vi "RT_stagectrl_readIFO_3levelramp_Nov4.vi"() -> ()   [LabVIEW 2019]
uses:
  <vilib>/Platform/TimedLoop/XDataNode/timing_clust.ctl
  <vilib>/Platform/TimedLoop/XDataNode/nitl_modes.ctl
  <vilib>/Platform/TimedLoop/XDataNode/wakeup.ctl
  <vilib>/FPGAPlugInAG/myRIO-1900/niLvFpga_Open_myRIO-1900.vi
  <vilib>/rvi/interface/common/dynamic/niFpgaDynamicAddResources.vi
  <vilib>/Utility/error.llb/Error Cluster From Error Code.vi
  <vilib>/rvi/errors/niLvFpgaAdjustHostInterfaceError.vi
  <vilib>/rvi/interface/nirviOpenFPGA/nirviOpenFPGA.xnode
  FPGA Bitfiles/studentchallenge_FPGATarget_FPGA1RADC1WDAC2A_R8uuw9uWLNg.lvbitx
  <vilib>/platform/TimedLoop/XDataNode/XDataNode.xnode
  <vilib>/rvi/interface/nirviReadWriteControl/nirviReadWriteControl.xnode
  NiFpgaLv.dll
  <vilib>/rvi/interface/Simulation/niFpgaSimulationCallBeginRW.vi
  <vilib>/Platform/TimedLoop/XDataNode/XDNodeRunTimeDep.lvlib
panel:
  in  "Stop":bool
  in  "P":dbl=2.0
  in  "I":dbl=0.005
  in  "D":dbl
  out "Control voltage":dbl=-0.4460961993175754 format="%#_3f"
  out "late?":bool
  out "?":cluster{"profile des(mm)":dbl, dbl, dbl}(graph)
  in  "Stage loop time (us)":i64=700
  out "Vp":dbl=-0.052695520808333285 format="%#_3g"
  out "Vi":dbl=0.4987253915842921 format="%#_3g"
  out "Vd":dbl format="%#_3g"
  out "profile des(mm)":dbl=1.6059943214036447
  in  "Profile track":bool
  in  "dt":i64=100
  in  "IFO loop time (us)":i64=70
  out "late? 2":bool
  out "IFO (um)":dbl
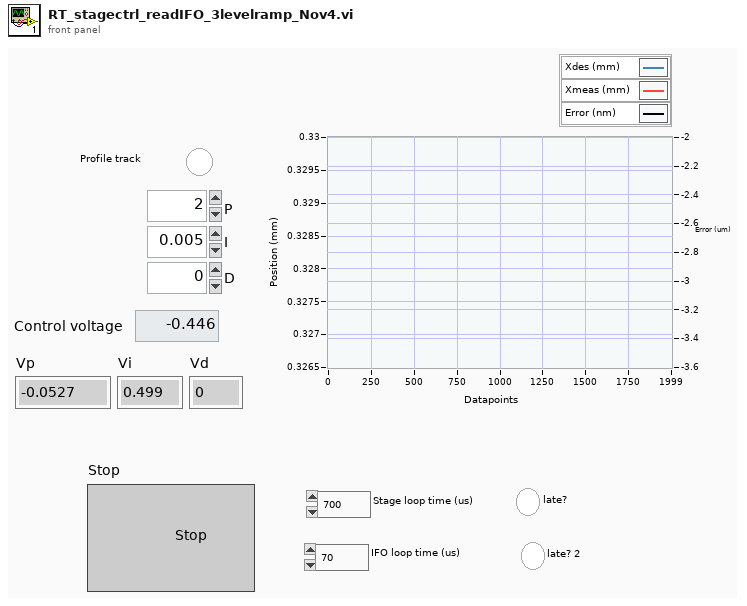
[diagram p1: front panel]
types:
  T1 = typedef "XDNodeRunTimeDep.lvlib/timing_clust.ctl" = cluster{"Expected End [f-1]":u64, "Actual End [f-1]":u64, "Finished Late? [f-1]":bool, "Expected End [i-1]":u64, "Actual End [i-1]":u64, "Finished Late? [i-1]":bool, "Expected Start [i]":u64, "Actual Start [i]":u64, "Expected Start [f]":u64, "Actual Start [f]":u64, "Source Name":string, "Structure Name":string, "Period":i64, "Deadline":i64, "Offset":i64, "Start":i64, "Priority":i32, "Timeout":i32, "Mode":T2, "Wakeup Reason":T3, "Error":errorcluster, "Source Type":string, "Secondary Source Type":string, "Global End Time":u64, "Global Start Time":u64, "Frame Duration":u64, "Iteration Duration":u64, "Assigned CPU":i32, "I/O Scan Engine Mode":u32}
  T2 = typedef "XDNodeRunTimeDep.lvlib/nitl_modes.ctl" = enum32{"No Change", "Process missed periods, maintain original phase", "Discard missed periods, maintain original phase", "Process missed periods, ignore original phase", "Discard missed periods, ignore original phase"}
  T3 = typedef "XDNodeRunTimeDep.lvlib/wakeup.ctl" = enum32{"Normal", "Aborted", "Asynchronous wakeup", "Timing source error", "Timed loop error", "Timeout"}
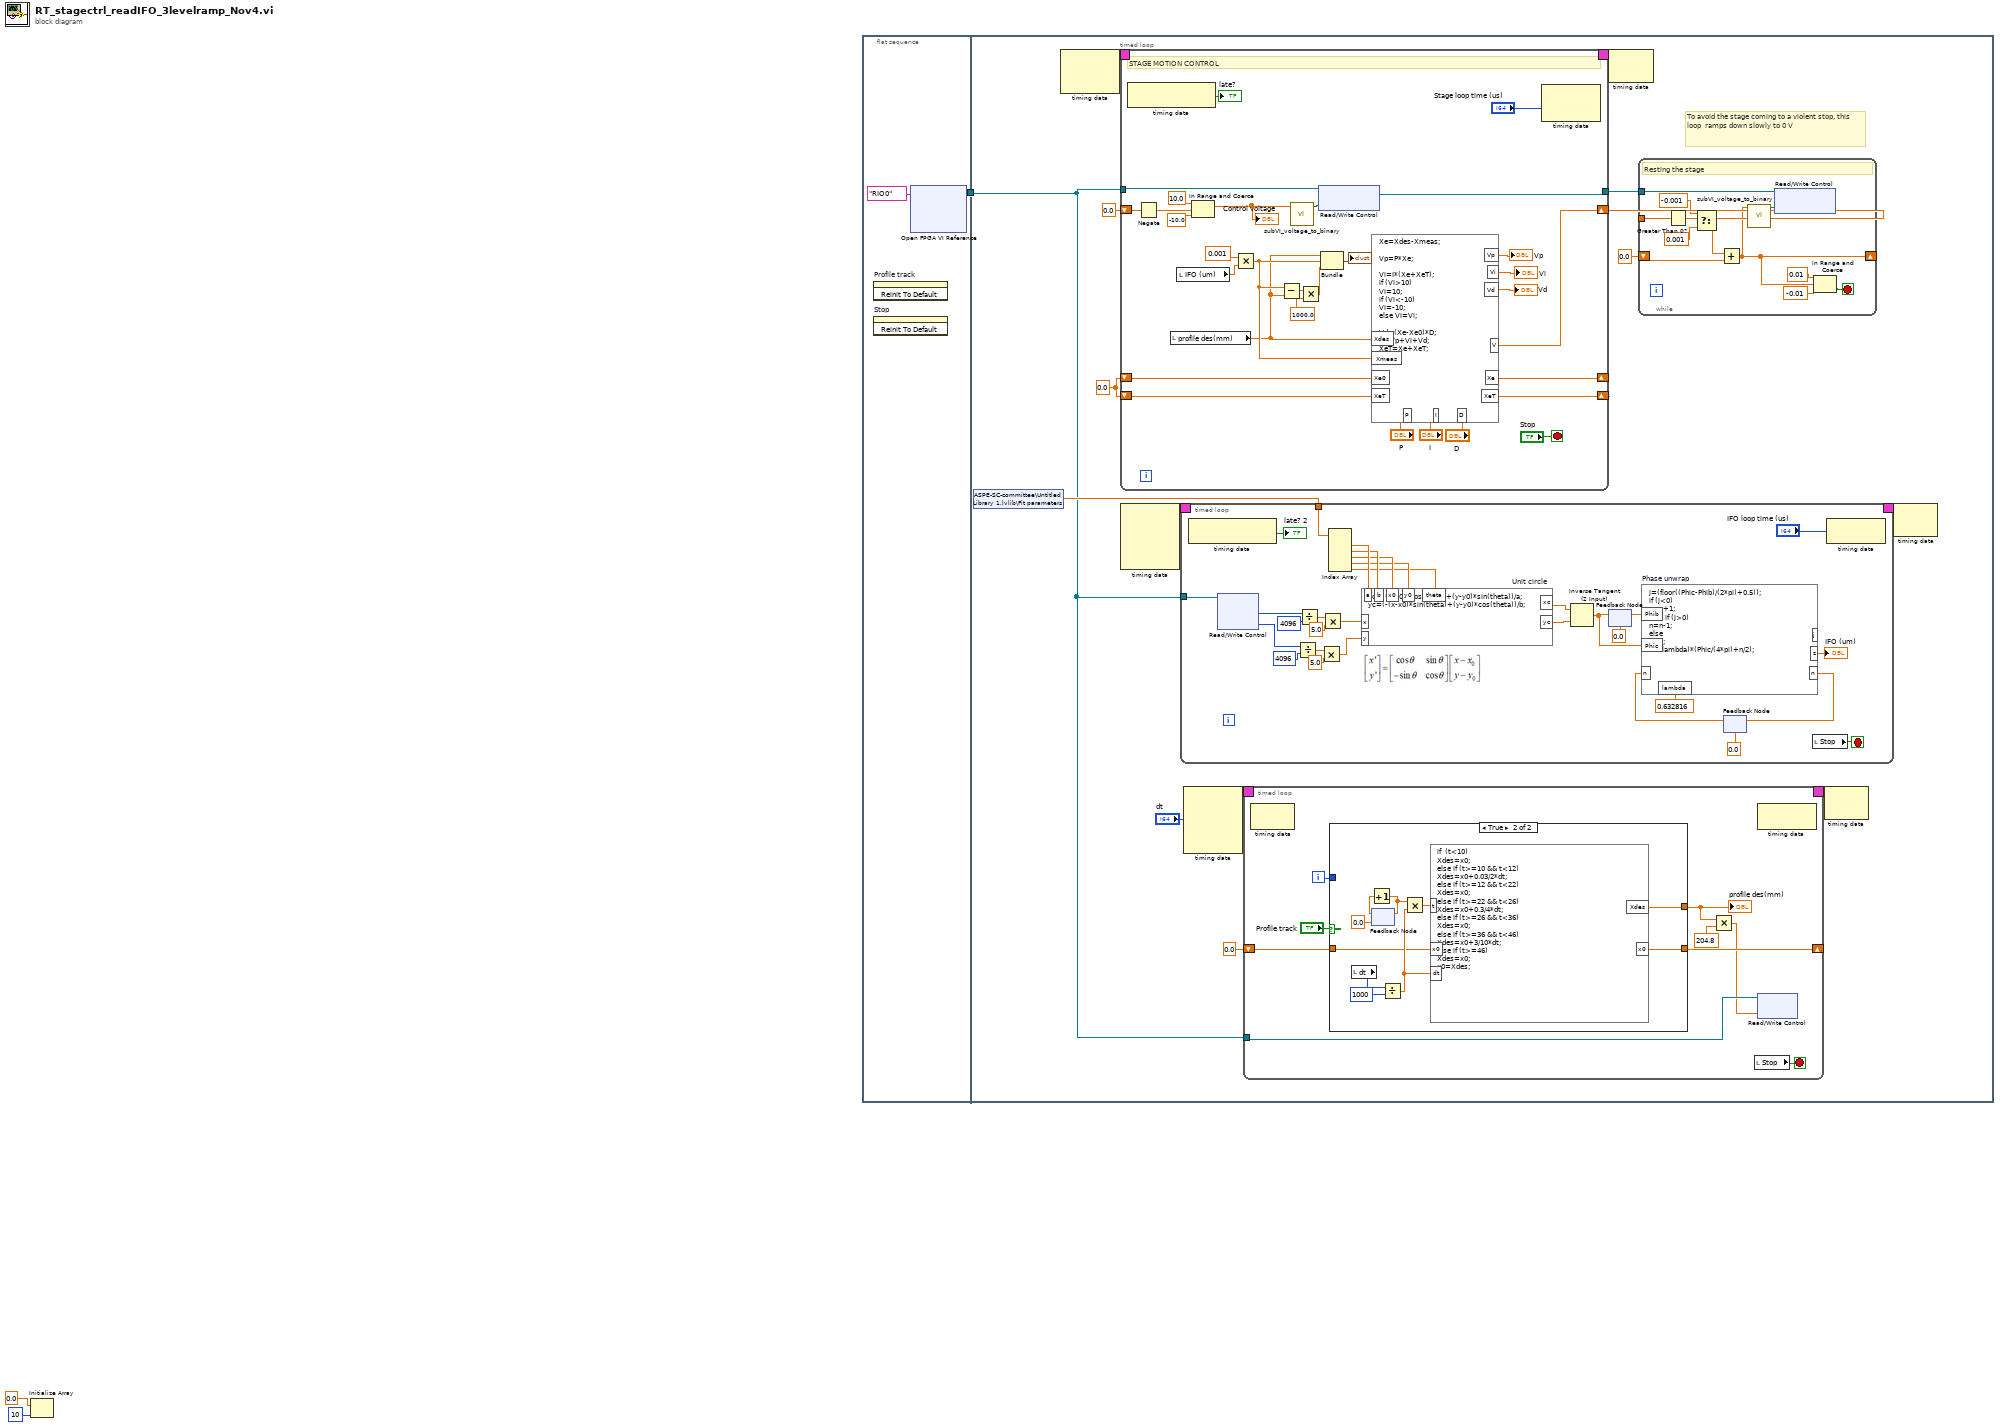
[diagram p0: block diagram]
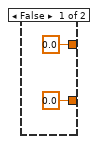
[diagram p2: hidden frame]
diagram:
  n1 = Initialize Array(0.0 ("element"), 10 ("dimension size")) -> ()  [unwired: 1 out]
  n2 = flat-sequence {
    tunnel: [w4] -> w1
    tunnel: w1 -> [w6]
    frame #0 {
      n3 = invoke on="Profile track" class="Bool (strict)" method="Reinit To Default"() -> ()  [unwired: 3 in, 3 out]
      n4 = invoke on="Stop" class="Bool (strict)" method="Reinit To Default"() -> ()  [unwired: 3 in, 3 out]
      n5 = xnode "Open FPGA VI Reference"("resource name"=tag "RIO0") -> ("FPGA VI Reference Out"=w4:refnum<k20>)  [unwired: 1 in, 1 out]
    }
    frame #1 {
      w13 = 0.0 ("Xe")
      # "To avoid the stage coming to a violent stop, this loop  ramps down slowly to 0 V"
      n6 = shared-variable "ASPE-SC-committee\\Untitled Library 1.lvlib\\Fit parameters"() -> (w10:dbl[])  [unwired: 1 in, 1 out]
      n7 = node-c288() -> (w20:T1)  [unwired: 2 in]
      n8 = timed-loop {
        timing: w20 -> [_]
        timing-out: [_] -> w19
        tunnel: [w114] -> w14
        tunnel: w6 -> [w101]
        shift-right: [w112] -> _
        shift-left: w13 -> [w111]
        shift-right: [w110] -> _
        shift-left: w13 -> [w109]
        shift-right: [w88] -> w9
        shift-left: 0.0 ("V") -> [w85]
        stop <- "Stop" stop-if-true
        # "STAGE MOTION CONTROL"
        n9 = node-c288() -> (→"late?":bool)  [unwired: 1 in]
        n10 = Negate(x=w85) -> (-x=w102:dbl)
        n11 = local read "profile des(mm)"() -> (w95:dbl)
        n12 = local read "IFO (um)"() -> (w99:dbl)
        n13 = In Range and Coerce(upper limit=10.0, x=w102, lower limit=-10.0) -> (coerced(x)=w86:dbl)  [unwired: 1 out]
        "Control voltage" <- w86
        n14 = Multiply(x=0.001, y=w99) -> (x*y=w96:dbl)
        n15 = Subtract(x=w96, y=w95) -> (x-y=w94:dbl)
        n16 = call "subVI_voltage_to_binary.vi"("voltage"=w86) -> ("binary"=w100:bool[])  [unwired: 10 in]
        n17 = Multiply(x=w94, y=1000.0) -> (x*y=w87:dbl)
        n18 = xnode "Read/Write Control"("FPGA VI Reference In"=w101, "DAC 1 write"=w100) -> ("FPGA VI Reference Out"=w114:refnum<k20>)  [unwired: 1 in, 1 out]
        n19 = Bundle("profile des(mm)"=w95, w96, w87) -> (→"?":cluster{"profile des(mm)":dbl, dbl, dbl})  [unwired: 1 in]
        n20 = formula code="Xe=Xdes-Xmeas;\n\nVp=P*Xe;\n\nVi=I*(Xe+XeT);\nif (Vi>10)\nVi=10;\nif (Vi<-10)\nVi=-10;\nelse Vi=Vi;\n\nVd=(Xe-Xe0)*D;\nV=Vp+Vi+Vd;\nXeT=Xe+XeT;"("Xdes"=w95, "Xmeas"=w96, "Xe0"=w111, "XeT"=w109, "P"="P", "I"="I", "D"="D") -> ("Xe"=w112:dbl, "V"=w88:dbl, "XeT"=w110:dbl, "Vp"=→"Vp":dbl, "Vi"=→"Vi":dbl, "Vd"=→"Vd":dbl)
        n21 = node-c288("Stage loop time (us)") -> ()  [unwired: 1 in, 1 out]
      }
      n22 = node-c288() -> (w16:T1)  [unwired: 4 in]
      n23 = timed-loop {
        timing: w16 -> [_]
        timing-out: [_] -> w15
        tunnel: w10 -> [w25]
        tunnel: w6 -> [w22]
        stop <- w23 stop-if-true
        n24 = node-c288() -> (→"late? 2":bool)  [unwired: 1 in]
        n25 = xnode "Read/Write Control"("FPGA VI Reference In"=w22) -> ("PD1"=w46:u16, "PD2"=w39:u16)  [unwired: 1 in, 2 out]
        n26 = Divide(x=w39, y=u16 4096) -> (x/y=w41:dbl)
        n27 = Divide(x=w46, y=u16 4096) -> (x/y=w44:dbl)
        n28 = Multiply(x=w41, y=5.0) -> (x*y=w37:dbl)
        n29 = Multiply(x=w44, y=5.0) -> (x*y=w42:dbl)
        n30 = Index Array(array=w25) -> (element #1=w36:dbl, element #2=w35:dbl, element #3=w34:dbl, element #4=w33:dbl, element #5=w32:dbl)  [unwired: 5 in]
        n31 = formula code="xc=((x-x0)*cos(theta)+(y-y0)*sin(theta))/a;\nyc=(-(x-x0)*sin(theta)+(y-y0)*cos(theta))/b;" "Unit circle"("a"=w36, "b"=w35, "x0"=w34, "y0"=w33, "theta"=w32, "x"=w42, "y"=w37) -> ("yc"=w49:dbl, "xc"=w50:dbl)
        n32 = Inverse Tangent (2 Input)(1:w49, 2:w50) -> (0:w28:dbl)
        n33 = feedback #1(0.0) -> (w29:dbl)
        n34 = feedback-in #1(w28) -> ()
        n35 = feedback #2(0.0 ("j")) -> (w30:dbl)
        n36 = formula code="j=(floor((Phic-Phib)/(2*pi)+0.5));\nif (j<0)\nn=n+1;\nelse if (j>0)\nn=n-1;\nelse\nn=n;\nz=(lambda)*(Phic/(4*pi)+n/2);" "Phase unwrap"("Phic"=w28, "Phib"=w29, "n"=w30, "lambda"=0.632816 ("input variable")) -> ("n"=w27:dbl, "z"=→"IFO (um)":dbl)  [unwired: 1 out]
        n37 = feedback-in #2(w27) -> ()
        n38 = local read "Stop"() -> (w23:bool)
        n39 = node-c288("IFO loop time (us)") -> ()  [unwired: 1 out]
      }
      n40 = node-c288("dt") -> (w18:T1)  [unwired: 3 in]
      n41 = timed-loop {
        timing: w18 -> [_]
        timing-out: [_] -> w17
        shift-right: [w66] -> _
        shift-left: 0.0 ("x0") -> [w65]
        tunnel: w6 -> [w61]
        i -> [w63]
        stop <- w62 stop-if-true
        n42 = node-c288() -> ()  [unwired: 1 in, 1 out]
        n43 = case shown="True" "Profile track" {
          tunnel: [0.0 ("x0") w75] -> w66
          tunnel: w65 -> [_ w74]
          tunnel: [0.0 ("Xdes") w69] -> w58
          tunnel: w63 -> [_ _]
          frame False {
          }
          frame True {
            n44 = local read "dt"() -> (w78:i64)
            n45 = feedback #3(0.0) -> (w71:dbl)
            n46 = Increment(x=w71) -> (x+1=w72:dbl)
            n47 = feedback-in #3(w72) -> ()
            n48 = Divide(x=w78, y=i64 1000) -> (x/y=w76:dbl)
            n49 = Multiply(x=w72, y=w76) -> (x*y=w73:dbl)
            n50 = formula code="if  (t<10)\nXdes=x0;\nelse if (t>=10 && t<12)\nXdes=x0+0.03/2*dt;\nelse if (t>=12 && t<22)\nXdes=x0;\nelse if (t>=22 && t<26)\nXdes=x0+0.3/4*dt;\nelse if (t>=26 && t<36)\nXdes=x0;\nelse if (t>=36 && t<46)\nXdes=x0+3/10*dt;\nelse if (t>=46)\nXdes=x0;\nx0=Xdes;"("t"=w73, "dt"=w76, "x0"=w74) -> ("Xdes"=w69:dbl, "x0"=w75:dbl)
          }
        }
        "profile des(mm)" <- w58
        n51 = Multiply(x=w58, y=204.8) -> (x*y=w59:dbl)
        n52 = local read "Stop"() -> (w62:bool)
        n53 = node-c288() -> ()  [unwired: 1 in, 1 out]
        n54 = xnode "Read/Write Control"("FPGA VI Reference In"=w61, "AO0"=w59) -> ()  [unwired: 1 in, 2 out]
      }
      n55 = node-c288(w19) -> ()  [unwired: 1 out]
      n56 = while {
        tunnel: w14 -> [w132]
        tunnel: w9 -> [w123]
        shift-right: [w122] -> _
        shift-left: 0.0 -> [w127]
        stop <- w124 stop-if-true
        # "Resting the stage"
        n57 = Greater Than 0?(x=w123) -> (x > 0?=w131:bool)
        n58 = Select(t=-0.001, s=w131, f=0.001) -> (s? t:f=w128:dbl)
        n59 = Add(x=w128, y=w127) -> (x+y=w122:dbl)
        n60 = call "subVI_voltage_to_binary.vi"("voltage"=w122) -> ("binary"=w133:bool[])  [unwired: 10 in]
        n61 = xnode "Read/Write Control"("FPGA VI Reference In"=w132, "DAC 1 write"=w133) -> ()  [unwired: 1 in, 2 out]
        n62 = In Range and Coerce(upper limit=0.01, x=w122, lower limit=-0.01) -> (In Range?=w124:bool)  [unwired: 1 out]
      }
      n63 = node-c288(w17) -> ()  [unwired: 1 out]
      n64 = node-c288(w15) -> ()  [unwired: 1 out]
    }
  }
